vi "readError.vi"(8 "error in (no error)":errorcluster, 10 "ErrorCode":i32, 11 "ElectrometerError in":refnum<class "ElectrometerError.lvclass">) -> (0 "error out":errorcluster, 2 "error":T1, 3 "ElectrometerError out":refnum<class "ElectrometerError.lvclass">)   [LabVIEW 2016, in "ElectrometerError.lvclass"]
uses:
  ElectrometerError.lvclass
  Controls/errorType.ctl
  ElectrometerError.lvclass/ElectrometerError.ctl
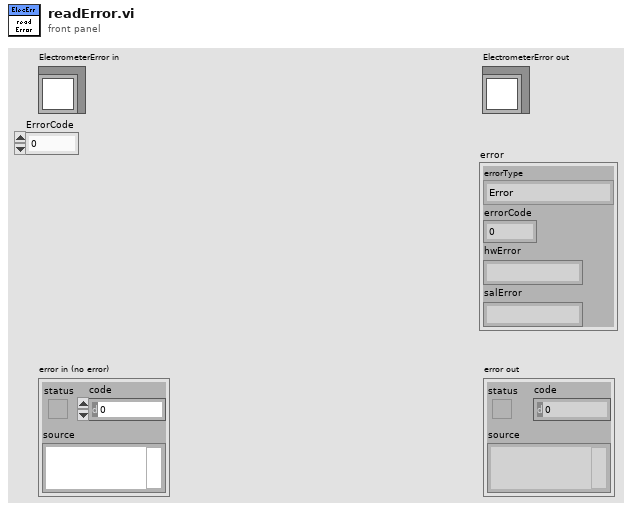
[diagram p1: front panel]
types:
  T1 = typedef "ElectrometerError.lvclass/errorType.ctl" = cluster{"errorType":enum16{"Error", "Warning", "None"}, "errorCode":dbl, "hwError":string, "salError":string}
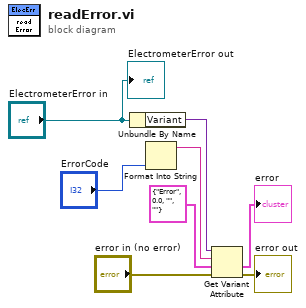
[diagram p0: block diagram]
diagram:
  n1 = Unbundle By Name("ElectrometerError in") -> ("Variant"=w7:variant)
  n2 = Format Into String("ErrorCode") -> (resulting string=w1:string)  [unwired: 3 in, 1 out]
  n3 = Get Variant Attribute(Variant=w7, name=w1, default value (empty Variant)=T1 {"errorType"=enum."Error", "errorCode"=0.0, "hwError"="", "salError"=""} ("error 2"), error in="error in (no error)") -> (value=→"error":T1, error out=→"error out":errorcluster)  [unwired: 2 out]
  "ElectrometerError out" <- "ElectrometerError in"
